vi "Register.vi"(11 "Template Event in":refnum<class "Template Event.lvclass">) -> (2 "Registration":refnum<event-registration>, 3 "Template Event out":refnum<class "Template Event.lvclass">)   [LabVIEW 2021, in "Template Event.lvlib" / "Template Event.lvclass"]
uses:
  Template Event.lvclass
  <vilib>/Nathan Davis/jettl/jettl/Msg Strategy/Msg Strategy.lvclass
  Template Event.lvclass/Template Event.ctl
  <vilib>/Nathan Davis/jettl/jettl/Event/Event.lvclass
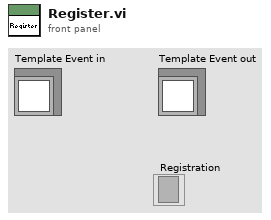
[diagram p1: front panel]
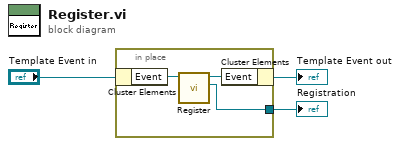
[diagram p0: block diagram]
diagram:
  n1 = in-place {
    in-place-border: [w4] -> w1
    n2 = in-place-cluster #1("Template Event in") -> ("Event"=w6:refnum<class "Event.lvclass">)
    n3 = call-dynamic "Register.vi"("Event in"=w6) -> ("Registration"=w4:refnum<event-registration>, "Event out"=w5:refnum<class "Event.lvclass">)  [unwired: 9 in]
    n4 = in-place-cluster #1("Event"=w5) -> (→"Template Event out":refnum<class "Template Event.lvclass">)
  }
  "Registration" <- w1
